vi "checkNumRows.vi"(0 "reference in":refnum<class "excelFile.lvclass">, 2 "Parts:":string[][](array[string]), 5 "error in (no error)":errorcluster) -> (14 "reference out":refnum<class "excelFile.lvclass">, 19 "error out":errorcluster)   [LabVIEW 2016, in "excelFile.lvclass"]
uses:
  excelFile.lvclass
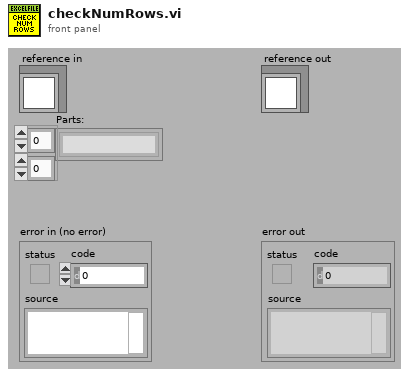
[diagram p1: front panel]
types:
  T1 = typedef "excelFile.lvclass/ObjectAttributesRef.ctl" = refnum<data-value>
  T2 = typedef "excelFile.lvclass/ObjectAttributes.ctl" = cluster{"MyAttribute":dbl, "path":string, "Refnum Excel":cluster{"Excel._Application":refnum<k7>, "Workbooks":refnum<k7>, "Open":refnum<k7>}, "data":string[][][], "save":bool, "fileType":T3, "rowsColor":u32[], "python_ref":refnum<class "python.lvclass">, "items_rows":i32[], "excel_range":i32[][], "TSR":cluster{"number":string, "TSR_path":path, "service_path":path, "email_to":string}, "excel_already_opened?":bool, "file_already_opened?":bool, "excel_protected_opened?":bool, "Refnum Cluster Worksheets":cluster{"Excel._Application":refnum<k7>, "Workbooks":refnum<k7>, "Open":refnum<k7>, "Worksheets":refnum<k7>, "Excel._Worksheet":refnum<k7>}, "#_rows_defective":i32, "#_rows_spare":i32}
  T3 = typedef "excelFile.lvclass/fileType.ctl" = enum16{"devices", "items", "partsTracking", "TSR"}
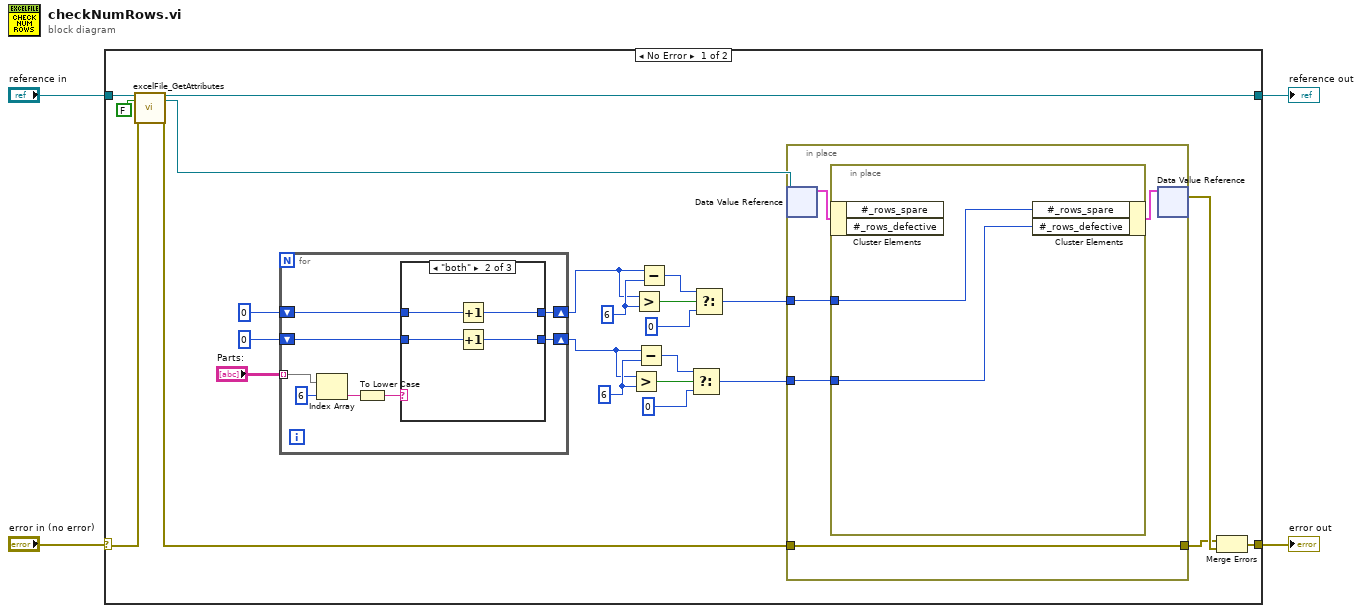
[diagram p0: block diagram]
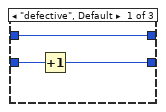
[diagram p2: hidden frame]
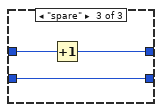
[diagram p3: hidden frame]
diagram:
  n1 = case shown="No Error" "error in (no error)" {
    selector: "error in (no error)" -> [w23 w55]
    tunnel: [w28 w55] -> w3
    tunnel: [w21 w54] -> w1
    tunnel: "reference in" -> [w25 w54]
    frame No Error {
      w9 = 6 ("y")
      w17 = 6 ("y")
      n2 = call "excelFile_GetAttributes.vi"("reference in"=w25, "return data? (T)"=FALSE, "error in (no error)"=w23) -> ("reference out"=w21:refnum<class "excelFile.lvclass">, "attributes ref"=w20:T1, "error out"=w22:errorcluster)  [unwired: 13 in, 1 out]
      n3 = for {
        tunnel: "Parts:" -> [w36] mode=indexing
        shift-right: [w30] -> w6
        shift-left: 0 ("y") -> [w32]
        shift-right: [w29] -> w11
        shift-left: 0 ("y") -> [w31]
        n4 = Index Array(array=w36, index=6) -> (element=w34:string)
        n5 = To Lower Case(string=w34) -> (all lower case string=w33:string)
        n6 = case shown="\"both\"" w33 {
          tunnel: w32 -> [w39 w43 w46]
          tunnel: w31 -> [w38 w42 w45]
          tunnel: [w39 w41 w44] -> w30
          tunnel: [w37 w40 w45] -> w29
          frame "defective", Default {
            n7 = Increment(x=w38) -> (x+1=w37:i32)
          }
          frame "both" {
            n8 = Increment(x=w43) -> (x+1=w41:i32)
            n9 = Increment(x=w42) -> (x+1=w40:i32)
          }
          frame "spare" {
            n10 = Increment(x=w46) -> (x+1=w44:i32)
          }
        }
      }
      n11 = Greater?(x=w11, y=w17) -> (0:w19:bool)
      n12 = Greater?(x=w6, y=w9) -> (0:w7:bool)
      n13 = Subtract(x=w11, y=w17) -> (x-y=w16:i32)
      n14 = Subtract(x=w6, y=w9) -> (x-y=w10:i32)
      n15 = Select(t=w16, s=w19, f=0 ("y")) -> (s? t:f=w15:i32)
      n16 = Select(t=w10, s=w7, f=0 ("y")) -> (s? t:f=w5:i32)
      n17 = in-place {
        in-place-border: w22 -> [w49]
        in-place-border: [w49] -> w26
        in-place-border: w15 -> [w48]
        in-place-border: w5 -> [w47]
        n18 = in-place-dvr #1(w20) -> (w50:T2)  [unwired: 1 out]
        n19 = in-place {
          in-place-border: w48 -> [w53]
          in-place-border: w47 -> [w52]
          n20 = in-place-cluster #2(w50) -> ()  [unwired: 2 out]
          n21 = in-place-cluster #2("#_rows_spare"=w52, "#_rows_defective"=w53) -> (w51:T2)
        }
        n22 = in-place-dvr #1(w51) -> (w27:errorcluster)  [unwired: 1 out]
      }
      n23 = Merge Errors(w26, w27) -> (w28:errorcluster)
    }
    frame Error {
    }
  }
  "error out" <- w3
  "reference out" <- w1
